vi "Mail.vi"(8 "error in (no error)":errorcluster caption="错误输入（无错误）", 10 "验证邮箱":T1, 11 "邮件信息":T2={"发送者地址"="csxcs_366@126.com", "发送者姓名"="", "接收者地址"=[], "邮件主题"="", "邮件内容"="", "添加附件"=[]}) -> (0 "error out":errorcluster caption="错误输出", 3 "MAIL 输出":refnum<class "Email.lvclass"> caption="DNL_LabVIEW Object out")   [LabVIEW 2012, in "Email.lvclass"]
uses:
  Email.lvclass
  MailInfo.ctl
  CredencialInfo.ctl
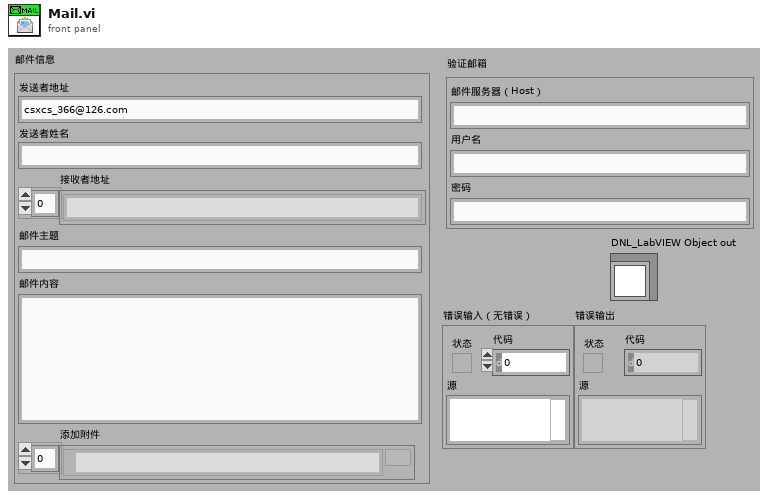
[diagram p1: front panel]
types:
  T1 = typedef "Email.lvclass/CredencialInfo.ctl" = cluster{"邮件服务器（Host）":string, "用户名":string, "密码":string}
  T2 = typedef "Email.lvclass/MailInfo.ctl" = cluster{"发送者地址":string, "发送者姓名":string, "接收者地址":string[], "邮件主题":string, "邮件内容":string, "添加附件":path[]}
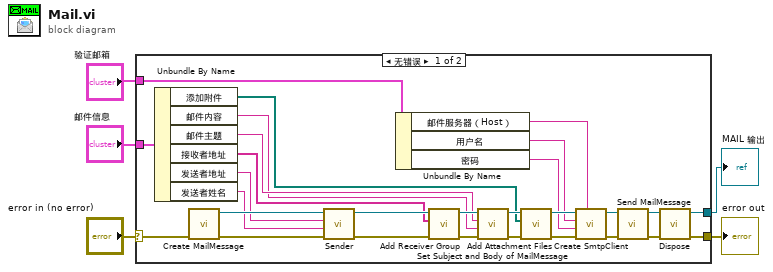
[diagram p0: block diagram]
diagram:
  n1 = case shown="无错误" "error in (no error)" {
    selector: "error in (no error)" -> [w32 w34]
    tunnel: [w19 w34] -> w4
    tunnel: [w20 _] -> w3
    tunnel: "邮件信息" -> [w17 _]
    tunnel: "验证邮箱" -> [w10 _]
    frame No Error {
      n2 = Unbundle By Name(w17) -> ("添加附件"=w11:path[], "邮件内容"=w12:string, "邮件主题"=w13:string, "接收者地址"=w14:string[], "发送者地址"=w16:string, "发送者姓名"=w15:string)
      n3 = call "Create MailMessage.vi"("error in (no error)"=w32) -> ("error out"=w31:errorcluster, "Email Out"=w33:refnum<class "Email.lvclass">)  [unwired: 9 in]
      n4 = call "Sender.vi"("error in (no error)"=w31, "Sender Name"=w15, "Sender Address"=w16, "Email In"=w33) -> ("error out"=w30:errorcluster, "Email Out"=w29:refnum<class "Email.lvclass">)  [unwired: 6 in]
      n5 = Unbundle By Name(w10) -> ("邮件服务器（Host）"=w9:string, "用户名"=w8:string, "密码"=w7:string)
      n6 = call "Add Receiver Group.vi"("error in (no error)"=w30, "Receiver Group"=w14, "Email In"=w29) -> ("error out"=w27:errorcluster, "Email Out"=w28:refnum<class "Email.lvclass">)  [unwired: 7 in]
      n7 = call "Set Subject and Body of MailMessage.vi"("error in (no error)"=w27, "Body"=w12, "Subject"=w13, "Email In"=w28) -> ("error out"=w25:errorcluster, "Email Out"=w26:refnum<class "Email.lvclass">)  [unwired: 6 in]
      n8 = call "Add Attachment Files.vi"("error in (no error)"=w25, "Attachment Files"=w11, "Email In"=w26) -> ("error out"=w24:errorcluster, "Email Out"=w18:refnum<class "Email.lvclass">)  [unwired: 7 in]
      n9 = call "Create SmtpClient.vi"("host"=w9, "error in (no error)"=w24, "password"=w7, "userName"=w8, "Email In"=w18) -> ("error out"=w23:errorcluster, "Email Out"=w6:refnum<class "Email.lvclass">)  [unwired: 5 in]
      n10 = call "Send MailMessage.vi"("error in (no error)"=w23, "Email In"=w6) -> ("error out"=w22:errorcluster, "Email out"=w21:refnum<class "Email.lvclass">)  [unwired: 8 in]
      n11 = call "Dispose.vi"("error in (no error)"=w22, "Mail 输入"=w21) -> ("error out"=w19:errorcluster, "Mail 输出"=w20:refnum<class "Email.lvclass">)  [unwired: 8 in]
    }
    frame Error {
    }
  }
  "error out" <- w4
  "MAIL 输出" <- w3
